vi "LSX Set Switch Active.vi"(6 "lAA":i32, 7 "lZA":i32, 8 "error in (no error)":errorcluster, 9 "lYA":i32, 10 "lXA":i32, 11 "lLSID":i32) -> (0 "error out":errorcluster, 3 "function return":i32)   [LabVIEW 2016, in "Tango_DLL.lvlib"]
doc: "TANGOAPI int TANGOCALL LSX_SetSwitchActive (int lLSID, int lXA, int lYA, int lZA, int lAA);"
uses:
  Tango_DLL.lvlib
  2017/Microscope Control/Device Library/Stages/Marzhauser/SCAN IM 120 x 80/Tango DLL VIs/Tango_DLL.dll
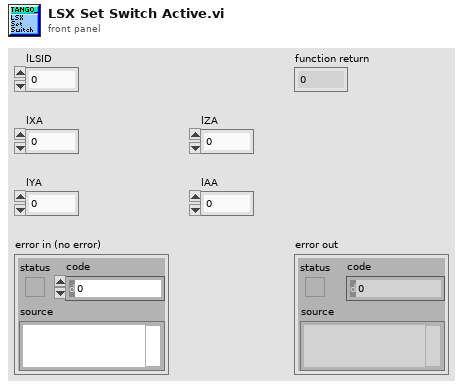
[diagram p1: front panel]
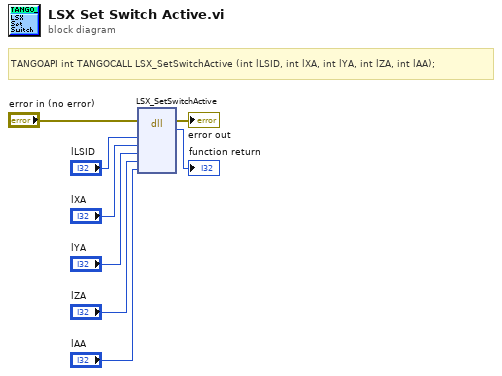
[diagram p0: block diagram]
diagram:
  # "TANGOAPI int TANGOCALL LSX_SetSwitchActive (int lLSID, int lXA, int lYA, int lZA, int lAA);"
  n1 = dll-call lib="C:/Users/4PiSMS/Documents/Microscope Control/2017/Microscope Control/Device Library/Stages/Marzhauser/SCAN IM 120 x 80/Tango DLL VIs/Tango_DLL.*" fn="LSX_SetSwitchActive"(error in="error in (no error)", "lLSID"="lLSID", "lXA"="lXA", "lYA"="lYA", "lZA"="lZA", "lAA"="lAA") -> (error out=→"error out":errorcluster, →"function return":i32)  [unwired: 7 in, 1 out]
